vi "tick_count.vi"() -> ()   [LabVIEW 2018]
panel:
  in  "Persistance":u8
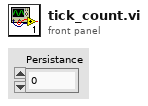
[diagram p1: front panel]
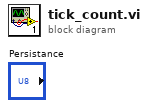
[diagram p0: block diagram]
diagram:
